vi "Report Results.vi"(5 "extra fields in":cluster{"skipped":bool, "skip reason":string}, 7 "pass in":bool, 8 "error in":errorcluster, 9 "unformatted test json out":string, 10 "test error in":errorcluster, 11 "vi ref in":refnum<vi>) -> (0 "error out":errorcluster, 2 "formatted test json out":string, 3 "ats json out":string)   [LabVIEW 2022 SP3]
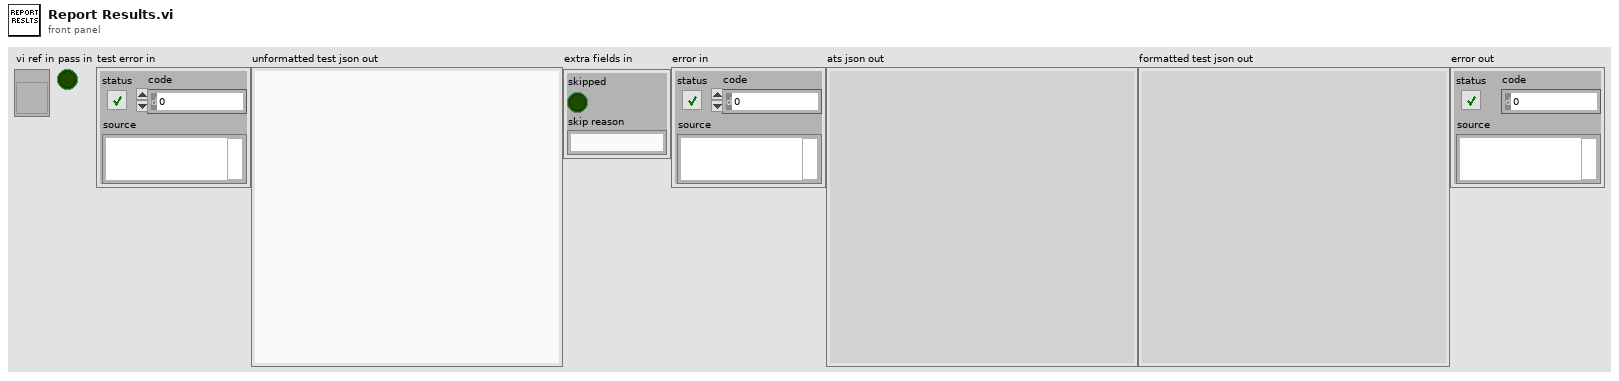
[diagram p1: front panel]
types:
  T1 = cluster{"ats json out":string, "test json out":string}
  T2 = cluster{"ats json out":string, "test json out":string}[]
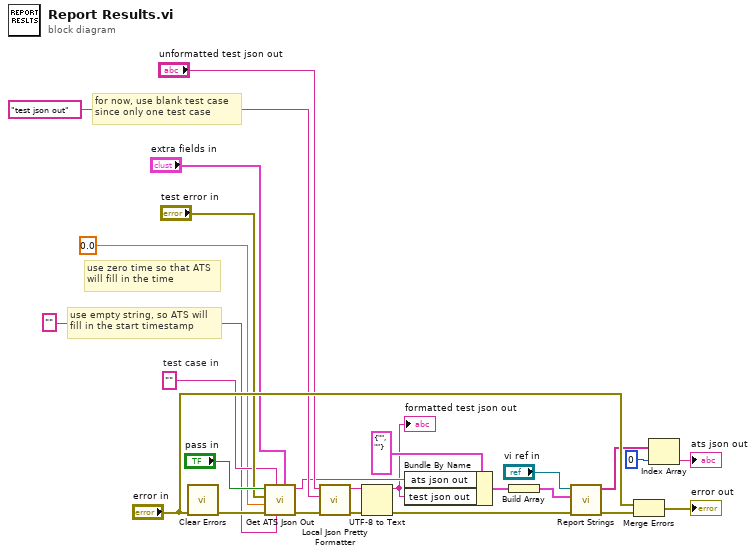
[diagram p0: block diagram]
diagram:
  w8 = ""  # test case in
  # "use empty string, so ATS will\nfill in the start timestamp"
  # "use zero time so that ATS\nwill fill in the time"
  # "for now, use blank test case\nsince only one test case"
  n1 = call <vilib>:"Clear Errors.vi"("error in (no error)"="error in") -> ("error out"=w21:errorcluster)  [unwired: 5 in, 1 out]
  n2 = call "Get ATS Json Out.vi"("extra fields in"="extra fields in", "start timestamp in"="", "test case in"=w8, "error in"=w21, "test time (s) in"=0.0, "test error in"="test error in", "pass in"="pass in") -> ("error out"=w18:errorcluster, "ats json out"=w13:string)  [unwired: 3 in]
  n3 = call "Local Json Pretty Formatter.vi"("error in"=w18, "data name in"="test json out", "json in"="unformatted test json out") -> ("error out"=w5:errorcluster, "json out"=w3:string)  [unwired: 7 in]
  n4 = UTF-8 to Text(8:w5, 11:w3) -> (0:w4:errorcluster, 3:w2:string)  [unwired: 1 in]
  "formatted test json out" <- w2
  n5 = Bundle By Name(cluster=T1 {"ats json out"="", "test json out"=""}, "ats json out"=w13, "test json out"=w2) -> (w14:T1)
  n6 = Build Array(w14) -> (w12:T2)
  n7 = call "Report Strings.vi"("error in"=w4, "data in"=w12, "vi ref in"="vi ref in") -> ("error out"=w23:errorcluster, "ats jsons out"=w10:string[])  [unwired: 6 in, 1 out]
  n8 = Merge Errors("error in", w23) -> (→"error out":errorcluster)
  n9 = Index Array(array=w10, index=0) -> (element=→"ats json out":string)
